vi "location of switch and scale.vi"() -> (0 "Scale":string, 3 "Switch":string)   [LabVIEW 2017]
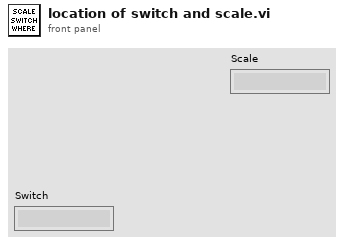
[diagram p1: front panel]
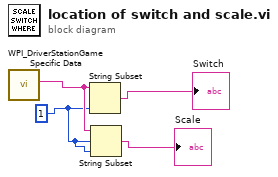
[diagram p0: block diagram]
diagram:
  w2 = 1
  n1 = call <vilib>:"WPI_DriverStationGame Specific Data.vi"() -> ("Game Specific Data"=w3:string)  [unwired: 11 in]
  n2 = String Subset(string=w3, length (rest)=w2) -> (substring=→"Switch":string)  [unwired: 1 in]
  n3 = String Subset(string=w3, offset (0)=w2, length (rest)=w2) -> (substring=→"Scale":string)
